vi "Globals.vi"() -> ()   [LabVIEW 2009, in "AMC.lvlib"]
uses:
  AMC.lvlib
panel:
  in  "Ack Message Name":string="AMC_Ack"
  in  "Default UDP Port":u16=54321
  in  "Dispatcher Process Name":string="AMC_Dispatch"
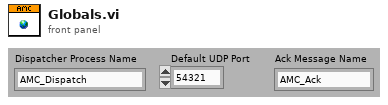
[diagram p1: front panel]
diagram:
